vi "Set Items (Label).vi"(6 "Items":refnum<class "IObject.lvclass">[](array[class]), 8 "error in (no error)":errorcluster, 10 "Label":string, 11 "MMI Scaling in":refnum<class "IObject.lvclass">) -> (0 "error out":errorcluster, 2 "Match?":bool, 3 "MMI Scaling out":refnum<class "IObject.lvclass">, 5 "Old items":refnum<class "IObject.lvclass">[](array[class]))   [LabVIEW 2013, in "IObject.lvclass"]
uses:
  IObject.lvclass
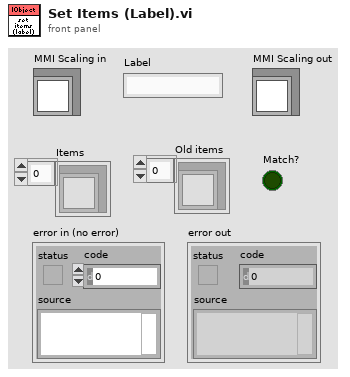
[diagram p1: front panel]
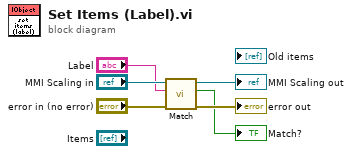
[diagram p0: block diagram]
diagram:
  n1 = call "Match.vi"("error in (no error)"="error in (no error)", "Label"="Label", "MMI Scaling in"="MMI Scaling in") -> ("error out"=→"error out":errorcluster, "Match?"=→"Match?":bool, "MMI Scaling out"=→"MMI Scaling out":refnum<class "IObject.lvclass">)  [unwired: 6 in]
